vi "4461 - Create Tasks AO.vi"(8 "error in (no error)":errorcluster, 11 "Instrument.Lockin in":refnum<class "Instrument.Lockin.lvclass">) -> (0 "error out":errorcluster, 3 "Instrument.Lockin out":refnum<class "Instrument.Lockin.lvclass">)   [LabVIEW 2016, in "Instrument.Lockin.lvclass"]
uses:
  Instrument.Lockin.lvclass
  Instrument.Lockin.lvclass/Instrument.Lockin.ctl
  <vilib>/DAQmx/create/channels.llb/DAQmx Create Channel (AO-Voltage-Basic).vi
  <resource>/objmgr/daqmx.rc
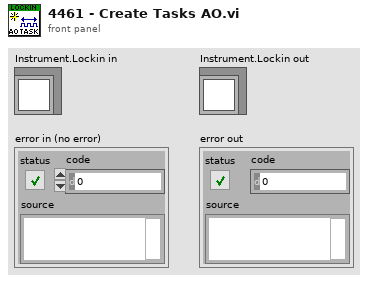
[diagram p1: front panel]
types:
  T1 = typedef "Instrument.Lockin.lvclass/AO.config-array.ctl" = T2[]
  T2 = typedef "Instrument.Lockin.lvclass/AO.config-cluster.ctl" = cluster{"AO.channels":tag, "AO.Range":T3, "output terminal configuration":i32, "DAQ Type":T4}
  T3 = typedef "Instrument.Lockin.lvclass/446xAO-enum.ctl" = enum16{"±0.1 V", "±1.0 V", "±10.0 V"}
  T4 = typedef "Instrument.Lockin.lvclass/DAQType-enum.ctl" = enum16{"None", "USB 4431", "PXI 446x"}
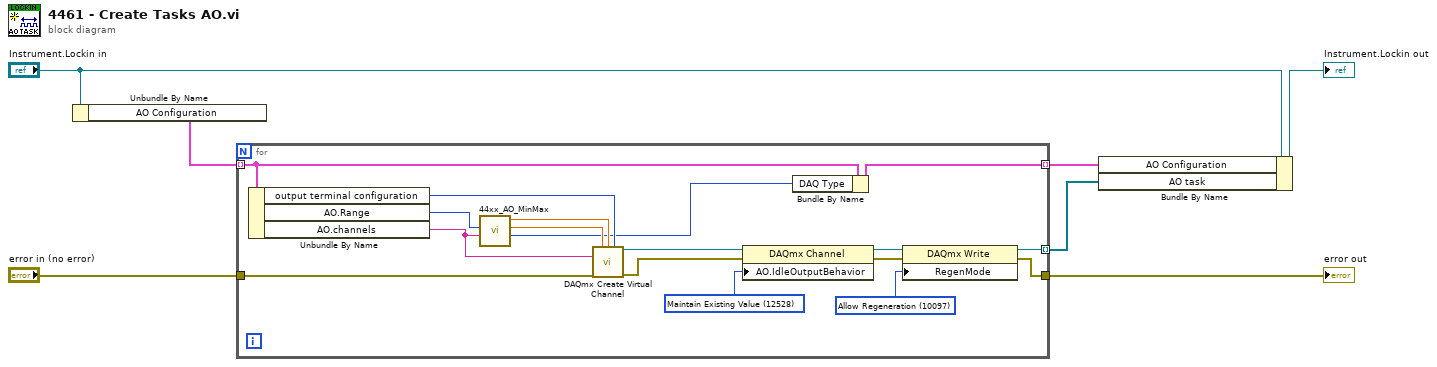
[diagram p0: block diagram]
diagram:
  n1 = Unbundle By Name("Instrument.Lockin in") -> ("AO Configuration"=w6:T1)
  n2 = for {
    tunnel: [w15] -> w1 mode=indexing
    tunnel: "error in (no error)" -> [w21]
    tunnel: [w9] -> w4
    tunnel: w6 -> [w8] mode=indexing
    tunnel: [w13] -> w3 mode=indexing
    w10 = 10097 items=["Allow Regeneration"=10097, "Do Not Allow Regeneration"=10158] ("RegenMode")
    w11 = 12528 items=["Zero Volts"=12526, "High-Impedance"=12527, "Maintain Existing Value"=12528] ("AO.IdleOutputBehavior")
    n3 = Unbundle By Name(w8) -> ("output terminal configuration"=w17:i32, "AO.Range"=w16:T3, "AO.channels"=w18:tag)
    n4 = call "44xx_AO_MinMax.vi"("AO.channels"=w18, "AO.Range"=w16) -> ("DAQ Type"=w14:T4, "AO.max"=w20:dbl, "AO.min"=w19:dbl)  [unwired: 7 in]
    n5 = call-poly <vilib>:"DAQmx Create Virtual Channel.vi"("maximum value"=w20, "minimum value"=w19, "output terminal configuration"=w17, "physical channels"=w18, "error in"=w21) -> ("task out"=w24:refnum<k21>, "error out"=w12:errorcluster)  [unwired: 9 in]
    n6 = property class="DAQmx Channel"(reference=w24, error in=w12, "AO.IdleOutputBehavior"=w11) -> (reference out=w23:refnum<k21>, error out=w22:errorcluster)
    n7 = Bundle By Name(cluster=w8, "DAQ Type"=w14) -> (w13:T2)
    n8 = property class="DAQmx Write"(reference=w23, error in=w22, "RegenMode"=w10) -> (reference out=w15:refnum<k21>, error out=w9:errorcluster)
  }
  "error out" <- w4
  n9 = Bundle By Name(cluster="Instrument.Lockin in", "AO Configuration"=w3, "AO task"=w1) -> (→"Instrument.Lockin out":refnum<class "Instrument.Lockin.lvclass">)
